vi "GetCurlSpeed.vi"(11 "SecondaryJoystickValues":dbl[](array[numeric])) -> (1 "Axis 4":dbl, 3 "Curl Speed":dbl)   [LabVIEW 2018]
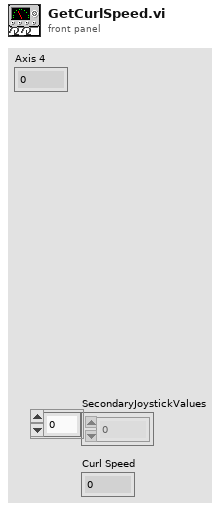
[diagram p1: front panel]
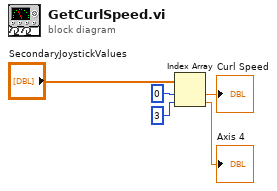
[diagram p0: block diagram]
diagram:
  n1 = Index Array(array="SecondaryJoystickValues", index #1=0 ("index"), index #2=3 ("index")) -> (element #1=→"Curl Speed":dbl, element #2=→"Axis 4":dbl)
